vi "SPI读写nodelay.vi"(2 "error in (no error)":errorcluster caption="错误输入（无错误）", 3 "从芯片读数据":string="spi r 0x04 0x0001", 4 "往芯片写数据":string="spi w 0x04 0x0001 0x01", 5 "VISA resource name":refnum<visa-resource-name>="COM3") -> (0 "error out":errorcluster, 1 "read buffer":string)   [LabVIEW 2015]
uses:
  <vilib>/Instr/_visa.llb/VISA Configure Serial Port (Instr).vi
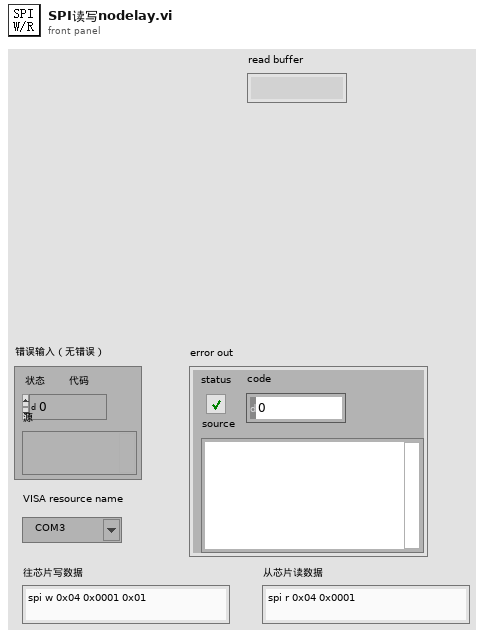
[diagram p1: front panel]
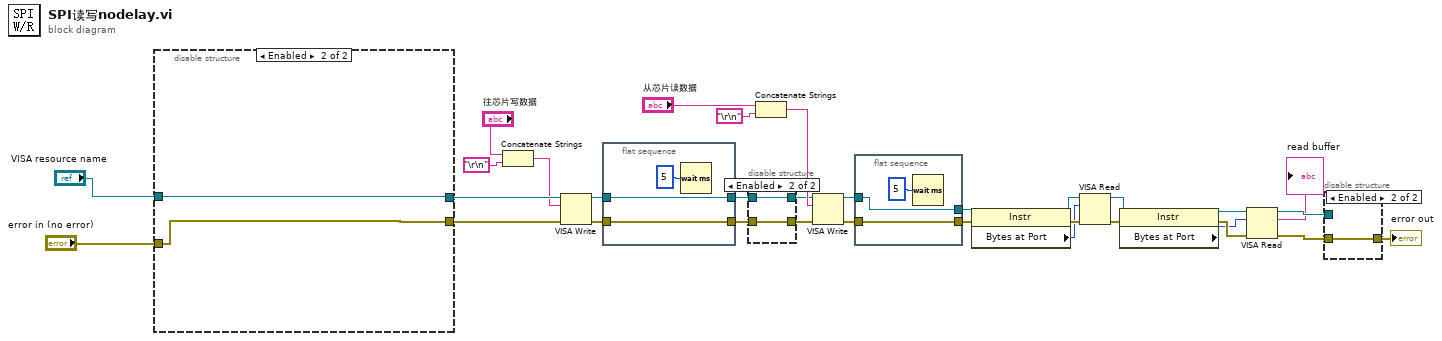
[diagram p0: block diagram]
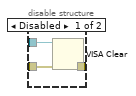
[diagram p2: hidden frame]
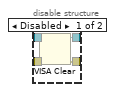
[diagram p3: hidden frame]
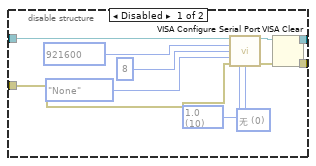
[diagram p4: hidden frame]
diagram:
  n1 = disable-structure shown="Enabled" {
    disable-tunnel: [w36 w44] -> w7
    disable-tunnel: [w35 w45] -> w4
    disable-tunnel: "VISA resource name" -> [w34 w45]
    disable-tunnel: "error in (no error)" -> [w33 w44]
    frame Disabled {
      w39 = u16 0 items=["无", "XON/XOFF", "RTS/CTS", "XON/XOFF & RTS/CTS", "DTR/DSR", "XON/XOFF & DTR/DSR"] ("flow control (0:none)")
      w40 = u16 10 items=["1.0"=10, "1.5"=15, "2.0"=20] ("stop bits (10: 1 bit)")
      n2 = call-poly "VISA Configure Serial Port"("VISA resource name"=w34, "baud rate (9600)"=u32 921600, "data bits (8)"=u16 8, "parity (0:none)"=enum16{"None", "Odd", "Even", "Mark", "Space"}."None", "error in (no error)"=w33, "stop bits (10: 1 bit)"=w40, "flow control (0:none)"=w39) -> ("VISA resource name out"=w38:refnum<visa-resource-name>, "error out"=w37:errorcluster)  [unwired: 7 in]
      n3 = VISA Clear(VISA resource name=w38, error in (no error)=w37) -> (VISA resource name out=w35:refnum<visa-resource-name>, error out=w36:errorcluster)
    }
    frame Enabled {
    }
  }
  n4 = Concatenate Strings("往芯片写数据", "\r\n") -> (w3:string)
  n5 = VISA Write(VISA resource name=w4, write buffer=w3, error in (no error)=w7) -> (VISA resource name out=w18:refnum<visa-resource-name>, error out=w17:errorcluster)  [unwired: 1 out]
  n6 = flat-sequence {
    tunnel: [w47] -> w13
    tunnel: w18 -> [w47]
    tunnel: [w46] -> w12
    tunnel: w17 -> [w46]
    frame #0 {
      n7 = Wait (ms)(milliseconds to wait=u32 5 ("等待时间（毫秒）")) -> ()  [unwired: 1 out]
    }
  }
  n8 = disable-structure shown="Enabled" {
    disable-tunnel: w13 -> [w52 w54]
    disable-tunnel: w12 -> [w51 w53]
    disable-tunnel: [w50 w54] -> w11
    disable-tunnel: [w49 w53] -> w2
    frame Disabled {
      n9 = VISA Clear(VISA resource name=w52, error in (no error)=w51) -> (VISA resource name out=w50:refnum<visa-resource-name>, error out=w49:errorcluster)
    }
    frame Enabled {
    }
  }
  n10 = Concatenate Strings("从芯片读数据", "\r\n") -> (w14:string)
  n11 = VISA Write(VISA resource name=w11, write buffer=w14, error in (no error)=w2) -> (VISA resource name out=w22:refnum<visa-resource-name>, error out=w21:errorcluster)  [unwired: 1 out]
  n12 = flat-sequence {
    tunnel: [w56] -> w32
    tunnel: w22 -> [w56]
    tunnel: [w55] -> w30
    tunnel: w21 -> [w55]
    frame #0 {
      n13 = Wait (ms)(milliseconds to wait=u32 5 ("等待时间（毫秒）")) -> ()  [unwired: 1 out]
    }
  }
  n14 = property class="Instr"(reference=w32, error in=w30) -> (reference out=w31:refnum<visa-resource-name>, error out=w29:errorcluster, "Bytes at Port"=w24:u32)
  n15 = VISA Read(VISA resource name=w31, byte count=w24, error in (no error)=w29) -> (VISA resource name out=w26:refnum<visa-resource-name>, error out=w25:errorcluster)  [unwired: 2 out]
  n16 = property class="Instr"(reference=w26, error in=w25) -> (reference out=w28:refnum<visa-resource-name>, error out=w27:errorcluster, "Bytes at Port"=w23:u32)
  n17 = VISA Read(VISA resource name=w28, byte count=w23, error in (no error)=w27) -> (VISA resource name out=w10:refnum<visa-resource-name>, read buffer=→"read buffer":string, error out=w8:errorcluster)  [unwired: 1 out]
  n18 = disable-structure shown="Enabled" {
    disable-tunnel: w10 -> [w60 _]
    disable-tunnel: [w59 w61] -> w9
    disable-tunnel: w8 -> [w58 w61]
    frame Disabled {
      n19 = VISA Clear(VISA resource name=w60, error in (no error)=w58) -> (error out=w59:errorcluster)  [unwired: 1 out]
    }
    frame Enabled {
    }
  }
  "error out" <- w9
